vi "Run.vi"(7 "Team Index":i32, 8 "Column":i32, 9 "Row":i32, 10 "View":i32[](array[numeric]) caption="View (Team Index, -1: empty)", 11 "64 In":refnum<class "64.lvclass">) -> (0 "Replicated":refnum<class "Square.lvclass">, 1 "Direction":T1, 2 "Action":T2, 3 "64 Out":refnum<class "64.lvclass">)   [LabVIEW 2015, in "64.lvclass"]
uses:
  64.lvclass
  Type Defs/Action Enum.ctl
  Type Defs/Direction Enum.ctl
  Square/Square.lvclass
  Formics/Attack Options.ctl
  SubVIs/Read-Only Globals.vi
  SubVIs/Globals (private).vi
  Common/Reverse Direction.vi
  Common/Common.lvlib
  Type Defs/SB Type Defs.lvlib
  Formics/Formics.lvclass
panel:
  # "NW\nN\nNE\nE\nSE\nS\nSW\nW"
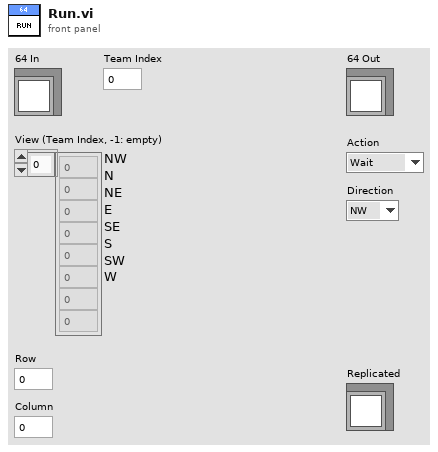
[diagram p1: front panel]
types:
  T1 = typedef "SB Type Defs.lvlib/Direction Enum.ctl" = enum16{"NW", "N", "NE", "E", "SE", "S", "SW", "W"}
  T2 = typedef "SB Type Defs.lvlib/Action Enum.ctl" = enum16{"Wait", "Move", "Attack", "Replicate"}
  T3 = typedef "Formics.lvclass/Attack Options.ctl" = enum16{"Attack", "Run", "Distract"}
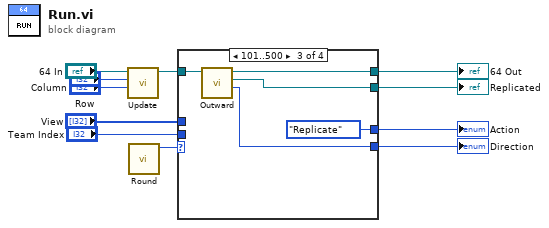
[diagram p0: block diagram]
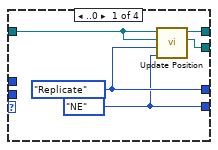
[diagram p2: hidden frame]
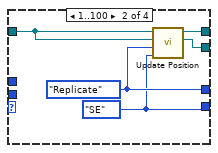
[diagram p3: hidden frame]
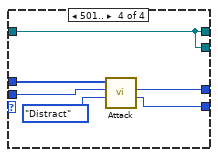
[diagram p4: hidden frame]
diagram:
  n1 = call "Update.vi"("Column"="Column", "Row"="Row", "64 in"="64 In") -> ("64 out"=w10:refnum<class "64.lvclass">)  [unwired: 8 in]
  n2 = call "Round.vi"() -> ("Round"=w3:i32)  [unwired: 11 in]
  n3 = case shown="101..500" w3 {
    tunnel: w10 -> [w15 w20 w26 w32]
    tunnel: [w14 w19 w25 w32] -> w6
    tunnel: [w16 w21 w24 w32] -> w7
    tunnel: [w13 w18 Action_Enum."Replicate" ("Action") w28] -> w5
    tunnel: [w12 w17 w23 w27] -> w4
    tunnel: "View" -> [_ _ _ w31]
    tunnel: "Team Index" -> [_ _ _ w30]
    frame ..0 {
      w12 = Direction_Enum."NE" ("Direction")
      w13 = Action_Enum."Replicate" ("Action")
      n4 = call "Update Position.vi"("Direction"=w12, "Action"=w13, "Replicated in"=w15, "64 in"=w15) -> ("Replicated out"=w16:refnum<class "64.lvclass">, "64 out"=w14:refnum<class "64.lvclass">)  [unwired: 6 in]
    }
    frame 1..100 {
      w17 = Direction_Enum."SE" ("Direction")
      w18 = Action_Enum."Replicate" ("Action")
      n5 = call "Update Position.vi"("Direction"=w17, "Action"=w18, "Replicated in"=w20, "64 in"=w20) -> ("Replicated out"=w21:refnum<class "64.lvclass">, "64 out"=w19:refnum<class "64.lvclass">)  [unwired: 6 in]
    }
    frame 101..500 {
      n6 = call "Outward.vi"("64 in"=w26) -> ("Direction"=w23:i32, "Replicated out"=w24:refnum<class "64.lvclass">, "64 out"=w25:refnum<class "64.lvclass">)  [unwired: 8 in]
    }
    frame 501.. {
      n7 = call "Attack.vi"("Attack?"=Attack_Options."Distract", "Team Index"=w30, "View"=w31) -> ("Direction"=w27:i32, "Action"=w28:T2)  [unwired: 3 in, 4 out]
    }
  }
  "64 Out" <- w6
  "Action" <- w5
  "Direction" <- w4
  "Replicated" <- w7
